vi "start.vi"(8 "error in (no error)":errorcluster, 11 "SpinCore in":refnum<class "SpinCore.lvclass">) -> (0 "error out":errorcluster, 3 "SpinCore out":refnum<class "SpinCore.lvclass">)   [LabVIEW 2009, in "Hardware.lvlib" / "Channels.lvlib" / "SpinCore.lvclass"]
uses:
  SpinCore.lvclass
  SpinCore.lvclass/SpinCore.ctl
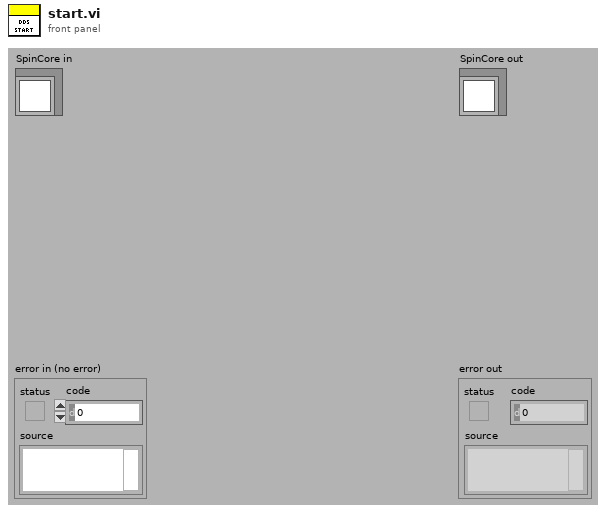
[diagram p1: front panel]
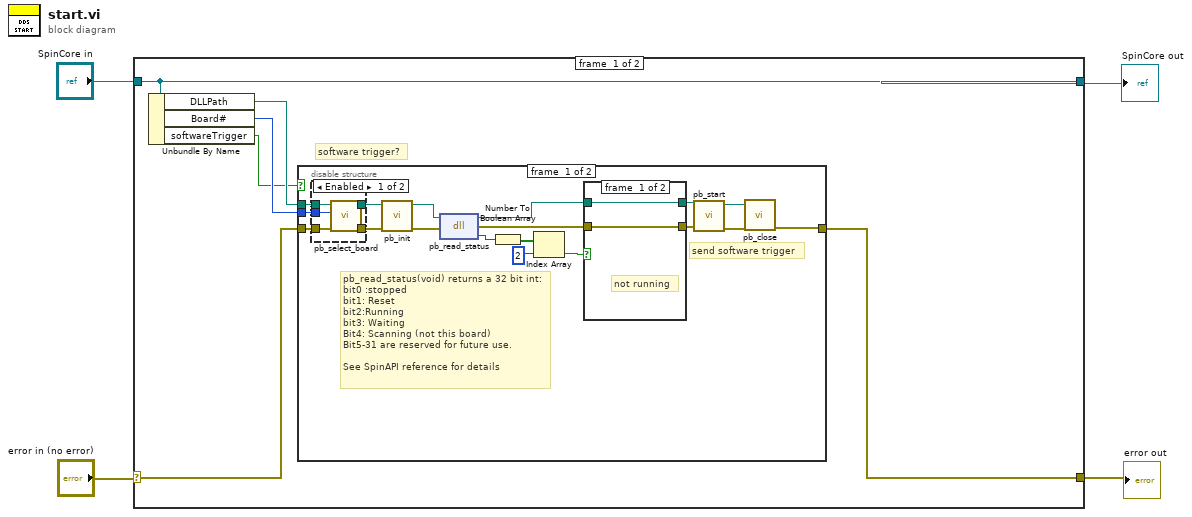
[diagram p0: block diagram]
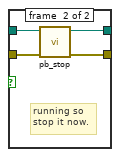
[diagram p3: hidden frame]
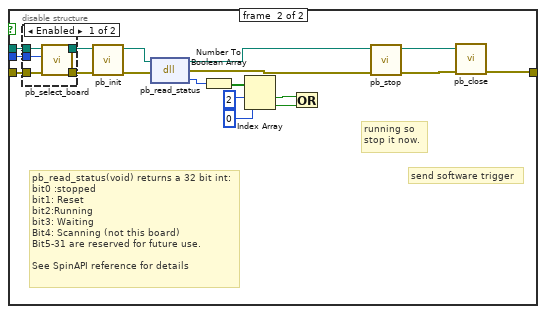
[diagram p4: hidden frame]
diagram:
  n1 = case shown="No Error" "error in (no error)" {
    selector: "error in (no error)" -> [w7 w67]
    tunnel: [w6 w67] -> w3
    tunnel: [w10 w68] -> w2
    tunnel: "SpinCore in" -> [w10 w68]
    frame #0 {
      # "software trigger?"
      n2 = Unbundle By Name(w10) -> ("DLLPath"=w9:path, "Board#"=w8:i32, "softwareTrigger"=w5:bool)
      n3 = case shown="False" w5 {
        tunnel: w9 -> [w24 w57]
        tunnel: w8 -> [w23 w56]
        tunnel: w7 -> [w22 w55]
        tunnel: [w21 w54] -> w6
        frame #0 {
          # "pb_read_status(void) returns a 32 bit int:\nbit0 :stopped\nbit1: Reset\nbit2:Running\nbit3: Waiting\nBit4: Scanning (not this board)\nBit5-31 are reserved for future use.\n\nSee SpinAPI reference for details"
          # "send software trigger"
          n4 = disable-structure shown="Enabled" {
            disable-tunnel: [w33 w34] -> w28
            disable-tunnel: [w32 w35] -> w27
            disable-tunnel: w24 -> [w31 w35]
            disable-tunnel: w23 -> [w30 _]
            disable-tunnel: w22 -> [w29 w34]
            frame #0 {
              n5 = call <userlib>:"pb_select_board.vi"("error in (no error)"=w29, "board_num"=w30, "path in"=w31) -> ("error out"=w33:errorcluster, "path out"=w32:path)  [unwired: 7 in]
            }
            frame #1 {
            }
          }
          n6 = call <userlib>:"pb_init.vi"("error in (no error)"=w28, "path in"=w27) -> ("error out"=w20:errorcluster, "path out"=w19:path)  [unwired: 8 in]
          n7 = dll-call lib="C:/Program Files/National Instruments/LabVIEW 2009/spinapi.dll" fn="pb_read_status"(path in=w19, error in=w20) -> (path out=w14:path, error out=w11:errorcluster, "status"=w18:i32)  [unwired: 1 in]
          n8 = Number To Boolean Array(number=w18) -> (Boolean array=w17:bool[])
          n9 = Index Array(array=w17, index=2) -> (element=w15:bool)
          n10 = case shown="True" w15 {
            tunnel: w14 -> [w37 w41]
            tunnel: [w37 w40] -> w13
            tunnel: [w36 w39] -> w12
            tunnel: w11 -> [w36 w38]
            frame #0 {
              # "not running"
            }
            frame #1 {
              # "running so \nstop it now."
              n11 = call <userlib>:"pb_stop.vi"("error in (no error)"=w38, "path in"=w41) -> ("error out"=w39:errorcluster, "path out"=w40:path)  [unwired: 8 in]
            }
          }
          n12 = call <userlib>:"pb_start.vi"("error in (no error)"=w12, "path in"=w13) -> ("error out"=w26:errorcluster, "path out"=w25:path)  [unwired: 8 in]
          n13 = call <userlib>:"pb_close.vi"("error in (no error)"=w26, "path in"=w25) -> ("error out"=w21:errorcluster)  [unwired: 8 in, 1 out]
        }
        frame #1 {
          # "running so \nstop it now."
          # "pb_read_status(void) returns a 32 bit int:\nbit0 :stopped\nbit1: Reset\nbit2:Running\nbit3: Waiting\nBit4: Scanning (not this board)\nBit5-31 are reserved for future use.\n\nSee SpinAPI reference for details"
          # "send software trigger"
          n14 = disable-structure shown="Enabled" {
            disable-tunnel: [w64 w65] -> w59
            disable-tunnel: [w63 w66] -> w58
            disable-tunnel: w57 -> [w62 w66]
            disable-tunnel: w56 -> [w61 _]
            disable-tunnel: w55 -> [w60 w65]
            frame #0 {
              n15 = call <userlib>:"pb_select_board.vi"("error in (no error)"=w60, "board_num"=w61, "path in"=w62) -> ("error out"=w64:errorcluster, "path out"=w63:path)  [unwired: 7 in]
            }
            frame #1 {
            }
          }
          n16 = call <userlib>:"pb_init.vi"("error in (no error)"=w59, "path in"=w58) -> ("error out"=w53:errorcluster, "path out"=w52:path)  [unwired: 8 in]
          n17 = dll-call lib="C:/Program Files/National Instruments/LabVIEW 2009/spinapi.dll" fn="pb_read_status"(path in=w52, error in=w53) -> (path out=w48:path, error out=w47:errorcluster, "status"=w51:i32)  [unwired: 1 in]
          n18 = Number To Boolean Array(number=w51) -> (Boolean array=w50:bool[])
          n19 = Index Array(array=w50, index #1=2, index #2=0) -> (element #1=w43:bool, element #2=w42:bool)
          n20 = Or(x=w43, y=w42) -> ()  [unwired: 1 out]
          n21 = call <userlib>:"pb_stop.vi"("error in (no error)"=w47, "path in"=w48) -> ("error out"=w45:errorcluster, "path out"=w46:path)  [unwired: 8 in]
          n22 = call <userlib>:"pb_close.vi"("error in (no error)"=w45, "path in"=w46) -> ("error out"=w54:errorcluster)  [unwired: 8 in, 1 out]
        }
      }
    }
    frame #1 {
    }
  }
  "error out" <- w3
  "SpinCore out" <- w2
